vi "LCDIO Get Chan Name.vi"(8 "error in (no error)":errorcluster caption="Fehler (Eingang, kein Fehler)", 11 "Channel Handle":i64) -> (0 "error out":errorcluster caption="Fehler (Ausgang)", 3 "Name":string)   [LabVIEW 2021, in "labbCAN_DigIO_API.lvlib"]
doc: "LCDIO_Func long LCDIO_CALL LCDIO_GetChanName(dev_hdl hChan,\n char *pNameStringBuf,\n int StringBufSize);"
uses:
  labbCAN_DigIO_API.lvlib
  labbCAN_DigIO_API.dll
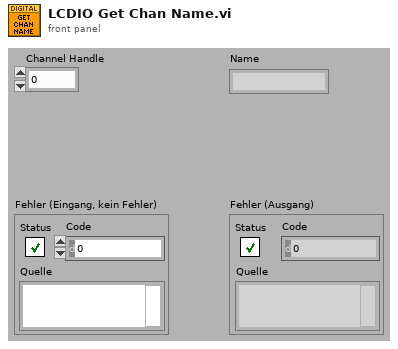
[diagram p1: front panel]
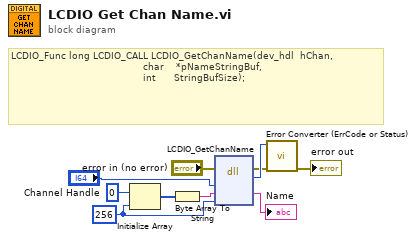
[diagram p0: block diagram]
diagram:
  w1 = 256 ("Dimension")
  # "LCDIO_Func long LCDIO_CALL LCDIO_GetChanName(dev_hdl  hChan,\n                                            char    *pNameStringBuf,\n                                            int      StringBufSize);"
  n1 = Initialize Array(u8 0 ("Element"), w1) -> (w9:u8[])
  n2 = Byte Array To String(unsigned byte array=w9) -> (string=w8:string)
  n3 = dll-call lib="C:/Users/olaja/AppData/Local/CETONI_SDK/labbCAN_DigIO_API.*" fn="LCDIO_GetChanName"(error in="error in (no error)", "Channel Handle"="Channel Handle", "Name"=w8, "StringBufSize"=w1) -> (error out=w3:errorcluster, "Rückgabetyp"=w4:i32, "Name"=→"Name":string)  [unwired: 4 in, 1 out]
  n4 = call "Error Converter (ErrCode or Status).vi"("error in (no error)"=w3, "error code"=w4) -> ("error out"=→"error out":errorcluster)  [unwired: 9 in]
